vi "MT Apply Pulse Shaping Filter (Generic).vi"(0 "symbols":cdb[](array[numeric]) format="%.2f", 5 "pulse shaping filter coefficients":dbl[](array[numeric]) format="%.2f", 7 "samples per symbol (16)":i32=16, 9 "symbol rate (Hz)":dbl=1.0, 11 "error in (no error)":errorcluster, 13 "reset? (T)":bool=TRUE) -> (4 "output complex waveform":T1={"t0"=0.0, "dt"=1.0, "Y"=[]} {"Y" format="%.3f"; "dt" format="%^.2e"; "t0" format="%.4f"}, 15 "error out":errorcluster)   [LabVIEW 2020, in "niDMT.lvlib"]
doc: "This polymorphic instance applies a pulse-shaping filter to an input stream comprised of PAM, ASK, QAM, and nonoffset PSK-modulated symbols. Separate polymorphic instances are available for offset PSK, FSK, and MSK."
uses:
  <vilib>/addons/Modulation/niDMT.lvlib
  <vilib>/addons/Modulation/Analog/controls/Complex Data Waveform.ctl
  <vilib>/addons/Modulation/niAMT.lvlib
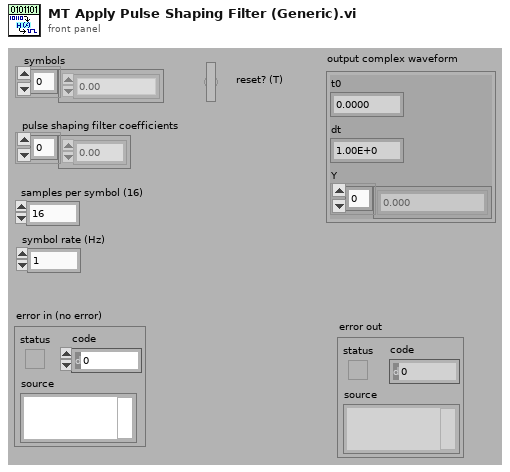
[diagram p1: front panel]
types:
  T1 = typedef "niAMT.lvlib/Complex Data Waveform.ctl" = cluster{"t0":dbl, "dt":dbl, "Y":cdb[]}
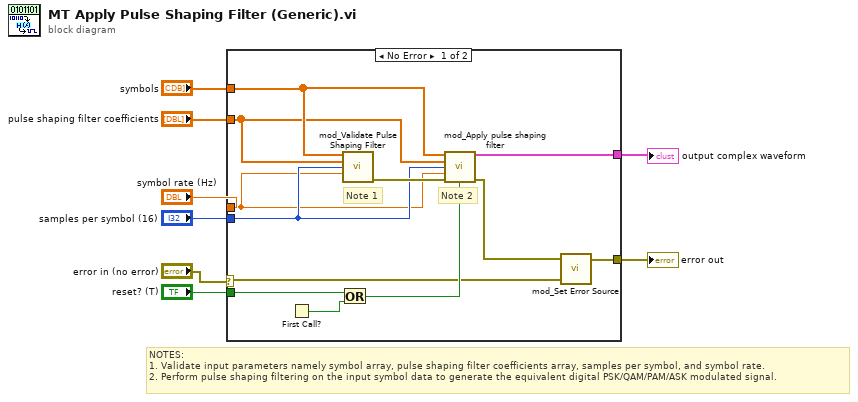
[diagram p0: block diagram]
diagram:
  # "NOTES:\n1. Validate input parameters namely symbol array, pulse shaping filter coefficients array, samples per symbol, and symbol rate.\n2. Perform pulse shaping filtering on the input symbol data to generate the equivalent digital PSK/QAM/PAM/ASK modulated signal."
  n1 = case shown="No Error" "error in (no error)" {
    selector: "error in (no error)" -> [w11 w21]
    tunnel: "symbols" -> [w15 _]
    tunnel: "pulse shaping filter coefficients" -> [w14 _]
    tunnel: "samples per symbol (16)" -> [w13 _]
    tunnel: "symbol rate (Hz)" -> [w12 _]
    tunnel: "reset? (T)" -> [w20 _]
    tunnel: [w9 w21] -> w2
    tunnel: [w17 _] -> w1
    frame No Error {
      # "Note 2"
      # "Note 1"
      n2 = First Call?() -> (First Call?: T/F=w19:bool)
      n3 = Or(x=w20, y=w19) -> (x .or. y?=w18:bool)
      n4 = call <vilib>:"mod_Validate Pulse Shaping Filter.vi"("symbols"=w15, "pulse shaping filter coefficients"=w14, "samples per symbol (16)"=w13, "symbol Rate, Hz"=w12) -> ("error out"=w16:errorcluster)  [unwired: 11 out]
      n5 = call <vilib>:"mod_Apply pulse shaping filter.vi"("symbols"=w15, "pulse shaping filter coefficients"=w14, "samples per symbol (16)"=w13, "symbol rate"=w12, "error in (no error)"=w16, "reset? (T)"=w18) -> ("output complex waveform"=w17:T1, "error out"=w10:errorcluster)  [unwired: 8 out]
      n6 = call <vilib>:"mod_Set Error Source.vi"("initial error in (no error)"=w11, "final error in (no error)"=w10) -> ("error out"=w9:errorcluster)  [unwired: 3 out]
    }
    frame Error {
    }
  }
  "error out" <- w2
  "output complex waveform" <- w1
